vi "For Loop.vi"() -> ()   [LabVIEW 2015, in "Simple Progress Bar.lvlib"]
uses:
  <vilib>/Utility/sysdir.llb/System Directory Type.ctl
  New Job Status.vi
  New Item Status.vi
  Class/Finish.vi
  Simple Progress Bar.lvlib
  Class/Bar.lvclass
panel:
  out "error out":errorcluster
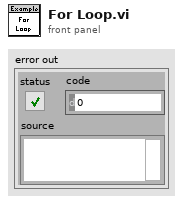
[diagram p1: front panel]
types:
  T1 = typedef "System Directory Type.ctl" = i32
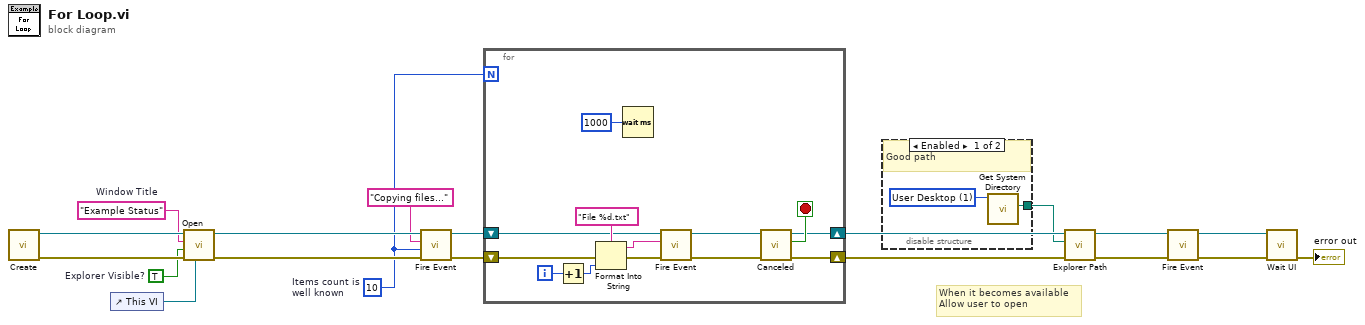
[diagram p0: block diagram]
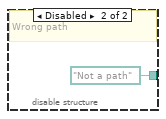
[diagram p2: hidden frame]
diagram:
  w7 = 10  # Items count is  well known
  w11 = "Example Status"  # Window Title
  w13 = TRUE  # Explorer Visible?
  # "When it becomes available\nAllow user to open"
  n1 = call "Create.vi"() -> ("error out"=w16:errorcluster, "Bar out"=w12:refnum<class "Bar.lvclass">)  [unwired: 10 in]
  n2 = control-ref of="This VI"() -> (w14:refnum<vi>)
  n3 = call "Open.vi"("VI"=w14, "error in (no error)"=w16, "Explorer Visible? (F)"=w13, "Window Title"=w11, "Bar in"=w12) -> ("error out"=w15:errorcluster, "Bar out"=w10:refnum<class "Bar.lvclass">)  [unwired: 5 in]
  n4 = call-poly "Fire Event.vi"("error in (no error)"=w15, "Items (unknown)"=w7, "Status"="Copying files...", "Bar in"=w10) -> ("error out"=w8:errorcluster, "Bar out"=w9:refnum<class "Bar.lvclass">)  [unwired: 6 in]
  n5 = for {
    N: w7 -> [_]
    shift-right: [w23] -> w18
    shift-left: w8 -> [w32]
    shift-right: [w20] -> w17
    shift-left: w9 -> [w26]
    i -> [w31]
    stop <- w22 stop-if-true
    n6 = Increment(x=w31) -> (x+1=w30:i32)
    n7 = Format Into String(format string="File %d.txt", error in=w32, w30) -> (resulting string=w25:string, error out=w27:errorcluster)  [unwired: 1 in]
    n8 = Wait (ms)(milliseconds to wait=u32 1000) -> ()  [unwired: 1 out]
    n9 = call-poly "Fire Event.vi"("error in (no error)"=w27, "Status"=w25, "Bar in"=w26) -> ("error out"=w24:errorcluster, "Bar out"=w21:refnum<class "Bar.lvclass">)  [unwired: 7 in]
    n10 = call "Canceled.vi"("error in (no error)"=w24, "Bar in"=w21) -> ("error out"=w23:errorcluster, "Canceled by user?"=w22:bool, "Bar out"=w20:refnum<class "Bar.lvclass">)  [unwired: 7 in]
  }
  n11 = disable-structure shown="Enabled" {
    disable-tunnel: [w33 path "Not a path" ("Explorer Path")] -> w5
    frame Enabled {
      w34 = T1 1 items=["User Home"=0, "User Desktop"=1, "User Documents"=2, "User Application Data"=3, "User Preferences"=4, "User Temporary"=5, "Public Documents"=6, "Public Application Data"=7, "Public Preferences"=8, "Public Cache"=13, "System Core Libraries"=9, "System Installed Libraries"=10, "Application Files"=11, "Boot Volume Root"=12] ("system directory type")
      # "Good path"
      n12 = call <vilib>:"Get System Directory.vi"("system directory type"=w34) -> ("system directory"=w33:path)  [unwired: 10 in]
    }
    frame Disabled {
      # "Wrong path"
    }
  }
  n13 = call "Explorer Path.vi"("error in (no error)"=w18, "Explorer Path"=w5, "Bar in"=w17) -> ("error out"=w3:errorcluster, "Bar out"=w4:refnum<class "Bar.lvclass">)  [unwired: 7 in]
  n14 = call-poly "Fire Event.vi"("error in (no error)"=w3, "Bar in"=w4) -> ("error out"=w1:errorcluster, "Bar out"=w2:refnum<class "Bar.lvclass">)  [unwired: 8 in]
  n15 = call "Wait UI.vi"("error in (no error)"=w1, "Bar in"=w2) -> ("error out"=→"error out":errorcluster)  [unwired: 6 in, 3 out]
